vi "hidSPD Close Session.vi"(8 "error in (no error)":errorcluster, 11 "deviceInfo in":string) -> (0 "error out":errorcluster, 3 "deviceInfo out":string)   [LabVIEW 2018, in "hidSPDLibForLabView.lvlib"]
uses:
  hidSPDLibForLabView.lvlib
  <vilib>/Utility/error.llb/Error Cluster From Error Code.vi
  <vilib>/ErrorRing/Error Ring.xnode
  hidSPD DLL files/libSPD.dll
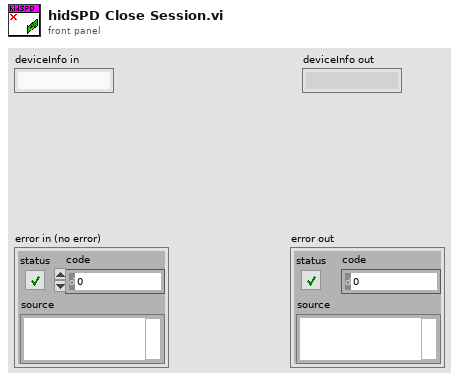
[diagram p1: front panel]
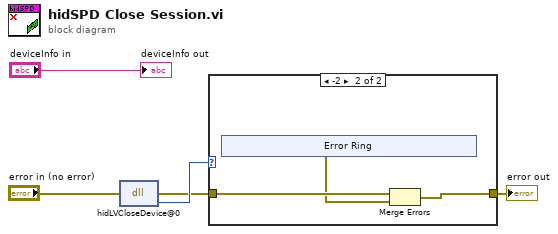
[diagram p0: block diagram]
diagram:
  n1 = dll-call lib="F:/NextCloud/SPD stand/Automative SPD Measurements/v 1.0.0/Instruments/SPD HID Interface/hidSPD DLL files/libSPD.dll" fn="hidLVCloseDevice@0"(error in="error in (no error)") -> (error out=w3:errorcluster, "return type"=w4:i32)  [unwired: 2 in, 1 out]
  n2 = case shown="-2" w4 {
    tunnel: w3 -> [w6 w9]
    tunnel: [w6 w7] -> w1
    frame 0, Default {
    }
    frame -2 {
      n3 = xnode "Error Ring"() -> ("error out"=w8:errorcluster)
      n4 = Merge Errors(w9, w8) -> (w7:errorcluster)
    }
  }
  "error out" <- w1
  "deviceInfo out" <- "deviceInfo in"
